vi "SetType.vi"(8 "error in (no error)":errorcluster, 10 "Type":string, 11 "Device in":refnum<class "Device.lvclass">) -> (0 "error out":errorcluster, 3 "Device out":refnum<class "Device.lvclass">)   [LabVIEW 2020, in "Device.lvlib" / "Device.lvclass"]
uses:
  Device.lvclass
  Device.lvclass/Device.ctl
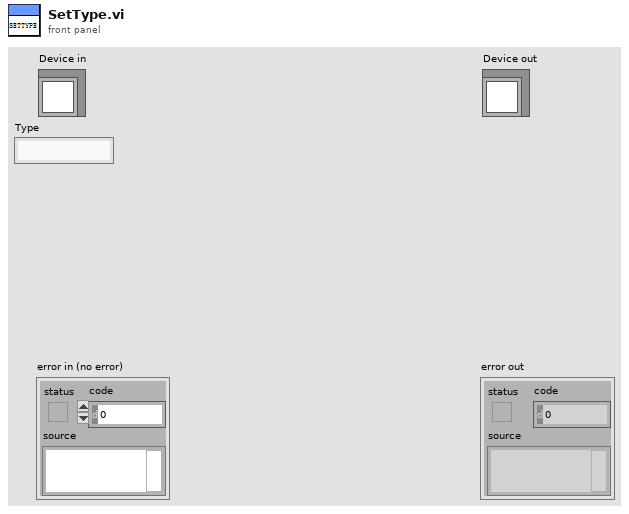
[diagram p1: front panel]
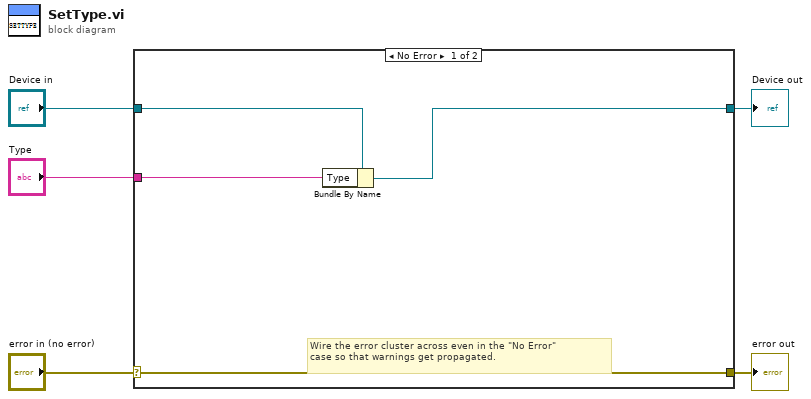
[diagram p0: block diagram]
diagram:
  n1 = case shown="No Error" "error in (no error)" {
    selector: "error in (no error)" -> [w9 w11]
    tunnel: [w9 w11] -> w4
    tunnel: [w6 w10] -> w2
    tunnel: "Device in" -> [w8 w10]
    tunnel: "Type" -> [w7 _]
    frame No Error {
      # "Wire the error cluster across even in the \"No Error\"\ncase so that warnings get propagated."
      n2 = Bundle By Name(cluster=w8, "Type"=w7) -> (w6:refnum<class "Device.lvclass">)
    }
    frame Error {
    }
  }
  "error out" <- w4
  "Device out" <- w2
